vi "Set Fast Kinetics.vi"(5 "vbin":i32, 6 "hbin":i32, 7 "mode":i32, 9 "time":sgl, 10 "seriesLength":i32, 11 "exposedRows":i32) -> (3 "function return":u32)   [LabVIEW 2018, in "Copy of Andor SDK.lvlib"]
doc: "EXPNETTYPE unsigned int WINAPI SetFastKinetics(int exposedRows, int seriesLength, float time, int mode, int hbin, int vbin);"
uses:
  Copy of Andor SDK.lvlib
  <userlib>/Andor SDK/ATMCD32D.dll
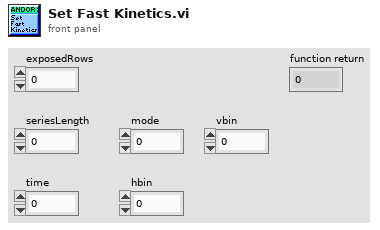
[diagram p1: front panel]
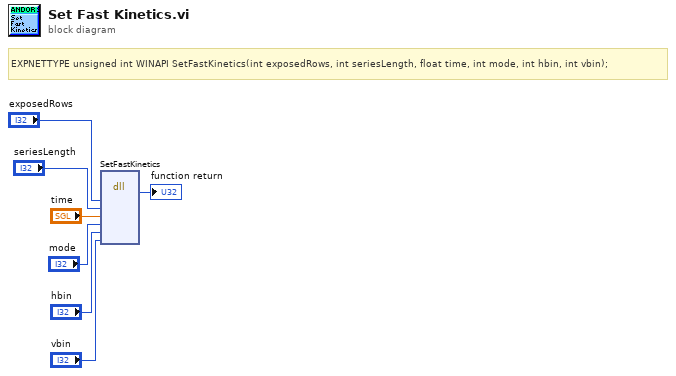
[diagram p0: block diagram]
diagram:
  # "EXPNETTYPE unsigned int WINAPI SetFastKinetics(int exposedRows, int seriesLength, float time, int mode, int hbin, int vbin);"
  n1 = dll-call lib="C:/Program Files (x86)/National Instruments/LabVIEW 2018/user.lib/Andor SDK/ATMCD32D.*" fn="SetFastKinetics"("exposedRows"="exposedRows", "seriesLength"="seriesLength", "time"="time", "mode"="mode", "hbin"="hbin", "vbin"="vbin") -> (→"function return":u32)  [unwired: 9 in, 2 out]
